vi "DP-Init Graph.vi"(0 "Nominal f2 SPL in":dbl[](array[numeric]), 5 "DP Freqs":T1[](array[typedef]), 7 "XYGraph in":refnum<vi>) -> (4 "Nominal f2 SPL out":dbl[](array[numeric]), 8 "XYGraph out":refnum<vi>, 14 "f2":dbl[](array[numeric]), 15 "plot vs freq":bool)   [LabVIEW 2020]
uses:
  Typedefs/DP-Freqs.ctl
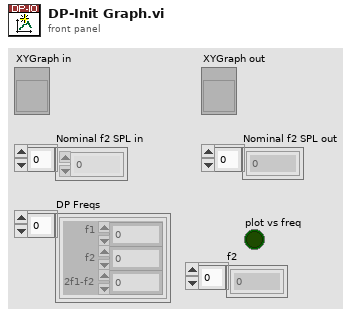
[diagram p1: front panel]
types:
  T1 = typedef "DP-Freqs.ctl" = cluster{"f1":dbl, "f2":dbl, "2f1-f2":dbl}
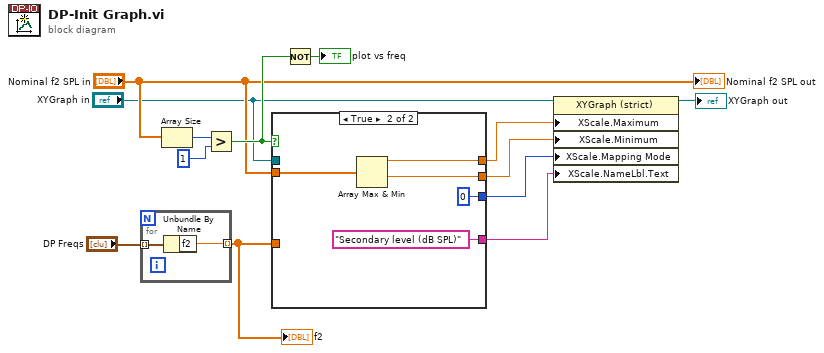
[diagram p0: block diagram]
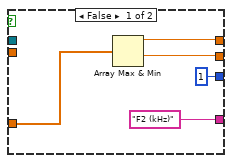
[diagram p2: hidden frame]
diagram:
  n1 = for {
    tunnel: "DP Freqs" -> [w15] mode=indexing
    tunnel: [w14] -> w8 mode=indexing
    n2 = Unbundle By Name(w15) -> ("f2"=w14:dbl)
  }
  "f2" <- w8
  n3 = Array Size(array="Nominal f2 SPL in") -> (size(s)=w13:i32)
  n4 = Greater?(x=w13, y=1) -> (0:w11:bool)
  n5 = case shown="True" w11 {
    tunnel: "Nominal f2 SPL in" -> [_ w25]
    tunnel: "XYGraph in" -> [_ _]
    tunnel: w8 -> [w20 _]
    tunnel: [w19 w24] -> w5
    tunnel: [w18 w23] -> w4
    tunnel: [u8 1 u8 0] -> w3
    tunnel: ["F2 (kHz)" "Secondary level (dB SPL)"] -> w2
    frame False {
      n6 = Array Max & Min(array=w20) -> (max value=w19:dbl, min value=w18:dbl)  [unwired: 2 out]
    }
    frame True {
      n7 = Array Max & Min(array=w25) -> (max value=w24:dbl, min value=w23:dbl)  [unwired: 2 out]
    }
  }
  n8 = Not(x=w11) -> (.not. x?=→"plot vs freq":bool)
  n9 = property class="XYGraph (strict)"(reference="XYGraph in", "XScale.Maximum"=w5, "XScale.Minimum"=w4, "XScale.Mapping Mode"=w3, "XScale.NameLbl.Text"=w2) -> (reference out=→"XYGraph out":refnum<vi>)  [unwired: 1 in, 1 out]
  "Nominal f2 SPL out" <- "Nominal f2 SPL in"
